vi "Get GUI items.vi"(0 "Run Block in":refnum<class "Run Block.lvclass">, 11 "error in (no error)":errorcluster) -> (4 "Run Block out":refnum<class "Run Block.lvclass">, 6 "Current RUN":T3, 8 "Schedule":T1 {"Number of cycles" min=1}, 10 "Skipped RUNs":T1 {"Number of cycles" min=1}, 15 "error out":errorcluster)   [LabVIEW 2020, in "Run Utilities.lvlib" / "Run Block.lvclass"]
doc: "Formats schedule, skipped RUNs and Current Run into GUI objects for display"
uses:
  Run Block.lvclass
  Run Instance/Run Instance - GUI.ctl
  Schedule/Array of Runs - GUI.ctl
  Cell/Cell - GUI.ctl
  Run Instance/Run Instance.lvclass
  Schedule/Schedule.lvclass
  Run Block.lvclass/Run Block.ctl
  Cell/Schedule Cell.lvclass
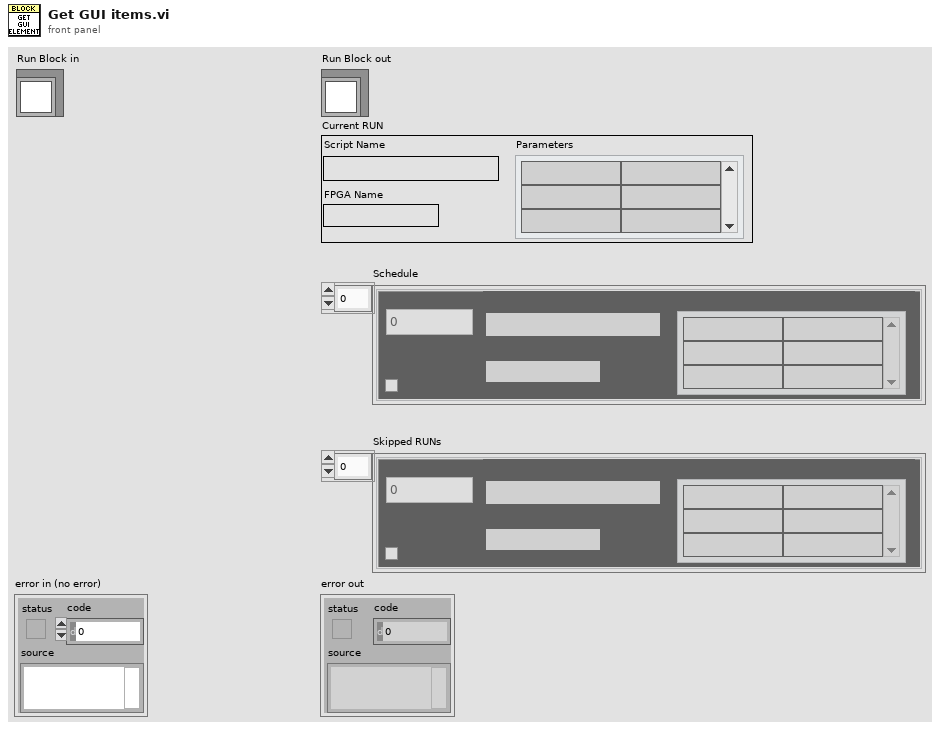
[diagram p1: front panel]
types:
  T1 = typedef "Run Utilities.lvlib/Schedule.lvclass/Array of Runs - GUI.ctl" = T2[]
  T2 = typedef "Run Utilities.lvlib/Schedule Cell.lvclass/Cell - GUI.ctl" = cluster{"Background Color":u32, "Number of cycles":u32, "Single RUN":T3, "Quality check":bool, "Cell Type":string}
  T3 = typedef "Run Utilities.lvlib/Run Instance.lvclass/Run Instance - GUI.ctl" = cluster{"Script Name":string, "Parameters":string[][], "FPGA Name":string}
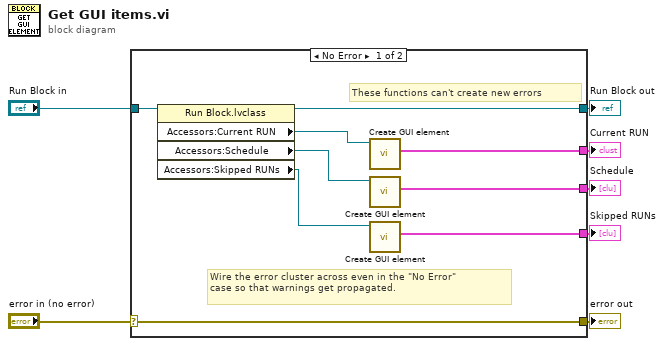
[diagram p0: block diagram]
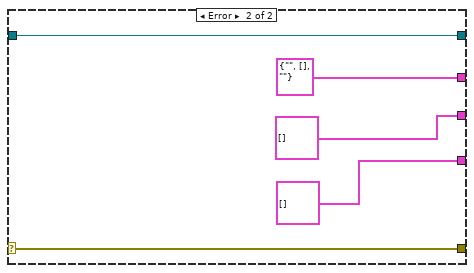
[diagram p2: hidden frame]
diagram:
  n1 = case shown="No Error" "error in (no error)" {
    selector: "error in (no error)" -> [w8 w21]
    tunnel: [w8 w21] -> w6
    tunnel: [w15 w20] -> w4
    tunnel: "Run Block in" -> [w16 w20]
    tunnel: [w11 T3 {"Script Name"="", "Parameters"=[], "FPGA Name"=""} ("Single RUN")] -> w3
    tunnel: [w10 T1 [] ("Array of Runs")] -> w2
    tunnel: [w9 T1 [] ("Array of Runs")] -> w1
    frame No Error {
      # "These functions can't create new errors"
      # "Wire the error cluster across even in the \"No Error\"\ncase so that warnings get propagated."
      n2 = property class="Run Block.lvclass"(reference=w16) -> (reference out=w15:refnum<class "Run Block.lvclass">, "Accessors:Current RUN"=w13:refnum<class "Run Instance.lvclass">, "Accessors:Schedule"=w14:refnum<class "Schedule.lvclass">, "Accessors:Skipped RUNs"=w12:refnum<class "Schedule.lvclass">)  [unwired: 1 in, 1 out]
      n3 = call-dynamic "Create GUI element.vi"("Run Instance in"=w13) -> ("Single RUN"=w11:T3)  [unwired: 8 in, 2 out]
      n4 = call-dynamic "Create GUI element.vi"("Schedule in"=w14) -> ("Array of Runs"=w10:T1)  [unwired: 8 in, 2 out]
      n5 = call-dynamic "Create GUI element.vi"("Schedule in"=w12) -> ("Array of Runs"=w9:T1)  [unwired: 8 in, 2 out]
    }
    frame Error {
    }
  }
  "error out" <- w6
  "Run Block out" <- w4
  "Current RUN" <- w3
  "Schedule" <- w2
  "Skipped RUNs" <- w1
